vi "LVPortFromObjectMap.vi"(8 "Allow Variant Values (f)":bool, 10 "Matlab Param Data":T1[](array[typedef]), 11 "Type (or value to update)":variant) -> (3 "Value":variant)   [LabVIEW 2017]
uses:
  LVPortObjectMapNamepathData.ctl
  LVPortObjectMapDataTypeEnum.ctl
  LVPortObjectMapContainerTypeEnum.ctl
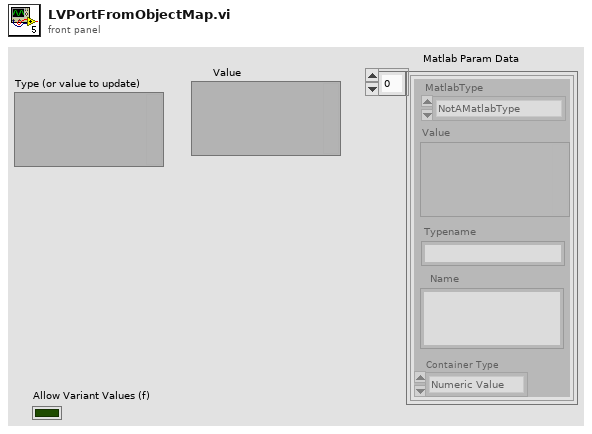
[diagram p1: front panel]
types:
  T1 = typedef "LVPortObjectMapNamepathData.ctl" = cluster{"MatlabType":T2, "Value":variant, "Name":string, "Typename":string, "Container Type":T3}
  T2 = typedef "LVPortObjectMapDataTypeEnum.ctl" = enum16{"NotAMatlabType", "Real", "Complex", "String", "Boolean"}
  T3 = typedef "LVPortObjectMapContainerTypeEnum.ctl" = enum16{"Numeric Value", "Numeric Array", "Waveform"}
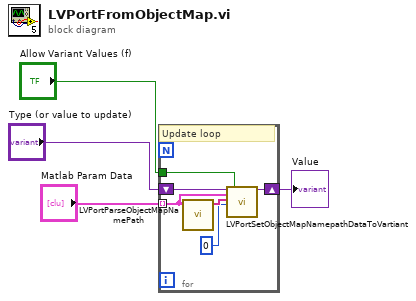
[diagram p0: block diagram]
diagram:
  n1 = for {
    tunnel: "Matlab Param Data" -> [w6] mode=indexing
    shift-right: [w8] -> w3
    shift-left: "Type (or value to update)" -> [w9]
    tunnel: "Allow Variant Values (f)" -> [w5]
    # "Update loop"
    n2 = call "LVPortParseObjectMapNamePath.vi"("MatlabDataBundle"=w6) -> ("Name parts array"=w10:string[])  [unwired: 10 in]
    n3 = call "LVPortSetObjectMapNamepathDataToVartiant.vi"("Type (or value to update)"=w9, "MatlabDataBundle"=w6, "NamePath"=w10, "Namepath Index"=0 ("curNameIndex"), "Allow Variant Values (f)"=w5) -> ("Value"=w8:variant)  [unwired: 13 in, 1 out]
  }
  "Value" <- w3
